vi "NISE.remote.Get Command Documentation.vi"(0 "SLSC Remote in":refnum<class "SLSC Interface.lvclass">, 5 "command":refnum<k21>, 11 "error in (no error)":errorcluster) -> (4 "SLSC Remote out":refnum<class "SLSC Interface.lvclass">, 6 "command out":refnum<k21>, 10 "Cmd.Doc":string, 15 "error out":errorcluster)   [LabVIEW 2016, in "SLSC Interface.lvclass"]
uses:
  SLSC Interface Class/SLSC Interface.lvclass
  SLSC Interface Class/SLSC Interface.lvclass/SLSC Interface.ctl
  SLSC Interface Class/NISE.Read client handle.vi
  SLSC Interface Class/NISE.Read URL.vi
  SLSC Interface Class/NISE.Read session.vi
  <vilib>/httpClient/POSTBuffer.vi
  <vilib>/NI/JSON Support for LabVIEW/JSON Value/Object/Get Value/Get Value (String).vi
  <vilib>/httpClient/LabVIEWHTTPClient.lvlib
  <vilib>/NI/JSON Support for LabVIEW/JSON Value/JSON Value.lvclass
  <vilib>/NI/NI JSONRPC Server Framework/Classes/Client/JSONRPC Client.lvclass
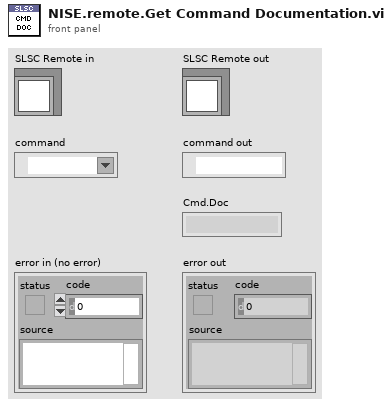
[diagram p1: front panel]
types:
  T1 = typedef "LabVIEWHTTPClient.lvlib/ClientHandle.ctl" = refnum<k1>
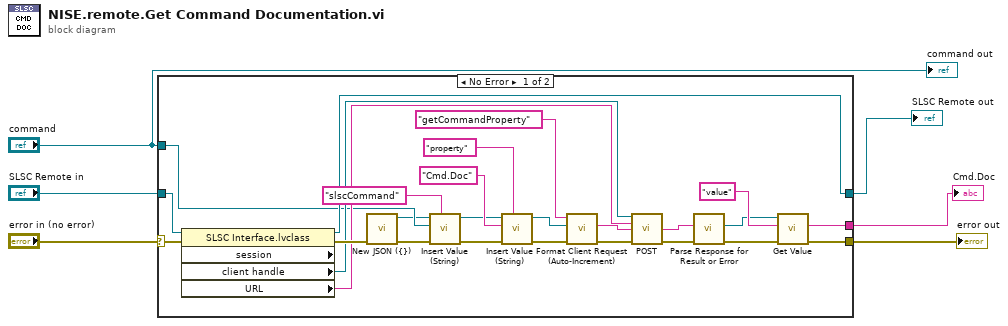
[diagram p0: block diagram]
diagram:
  n1 = case shown="No Error" "error in (no error)" {
    selector: "error in (no error)" -> [w30 w33]
    tunnel: "SLSC Remote in" -> [w32 w34]
    tunnel: [w31 w34] -> w3
    tunnel: [w20 w33] -> w1
    tunnel: [w19 _] -> w2
    tunnel: "command" -> [w12 _]
    frame No Error {
      n2 = property class="SLSC Interface.lvclass" props=["session", "client handle", "URL"](reference=w32, error in=w30) -> (reference out=w31:refnum<class "SLSC Interface.lvclass">, error out=w29:errorcluster, "client handle"=w25:T1, "URL"=w24:string)  [unwired: 1 out]
      n3 = call <vilib>:"New JSON ({}).vi"("error in (no error)"=w29) -> ("error out"=w28:errorcluster, "JSON Value out"=w9:refnum<class "JSON Value.lvclass">)  [unwired: 9 in]
      n4 = call <vilib>:"Insert Value (String).vi"("key"="slscCommand" ("Name"), "error in (no error)"=w28, "value"=w12, "JSON Value in"=w9) -> ("error out"=w15:errorcluster, "JSON Value out"=w8:refnum<class "JSON Value.lvclass">)  [unwired: 5 in, 1 out]
      n5 = call <vilib>:"Insert Value (String).vi"("key"="property" ("Name"), "error in (no error)"=w15, "value"="Cmd.Doc" ("String"), "JSON Value in"=w8) -> ("error out"=w17:errorcluster, "JSON Value out"=w18:refnum<class "JSON Value.lvclass">)  [unwired: 5 in, 1 out]
      n6 = call <vilib>:"Format Client Request (Auto-Increment).vi"("error in (no error)"=w17, "JSON Value in"=w18, "method"="getCommandProperty") -> ("error out"=w23:errorcluster, "Request String"=w26:string)  [unwired: 7 in]
      n7 = call-poly <vilib>:"POST.vi"("client handle"=w25, "url"=w24, "buffer"=w26, "error in (no error)"=w23) -> ("body"=w22:string, "error out"=w21:errorcluster)  [unwired: 8 in, 2 out]
      n8 = call <vilib>:"Parse Response for Result or Error.vi"("error in"=w21, "Response String In"=w22) -> ("error out"=w14:errorcluster, "JSON Value out"=w7:refnum<class "JSON Value.lvclass">)  [unwired: 7 in, 1 out]
      n9 = call-poly <vilib>:"Get Value.vi"("error in (no error)"=w14, "key"="value" ("Parameter Name"), "JSON Value in"=w7) -> ("error out"=w20:errorcluster, "value"=w19:string)  [unwired: 7 in]
    }
    frame Error {
    }
  }
  "error out" <- w1
  "SLSC Remote out" <- w3
  "Cmd.Doc" <- w2
  "command out" <- "command"
